vi "Fire Refresh Markers.vi"(8 "error in (no error)":errorcluster, 11 "SequenceViewPanel in":refnum<class "SequenceViewPanel.lvclass">) -> (0 "error out":errorcluster, 3 "SequenceViewPanel out":refnum<class "SequenceViewPanel.lvclass">)   [LabVIEW 2020, in "TSnax UI.lvlib" / "SequenceViewPanel.lvclass"]
uses:
  SequenceViewPanel.lvclass
  SequenceViewPanel.lvclass/SequenceViewPanel.ctl
  3c1a44d5-48fc-4b93-aa61-ebc8600dc4e9.vi
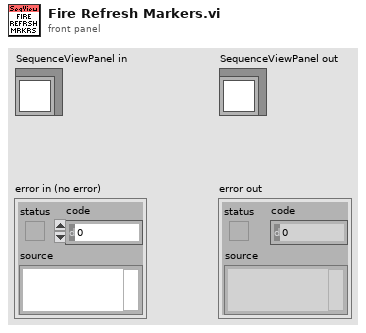
[diagram p1: front panel]
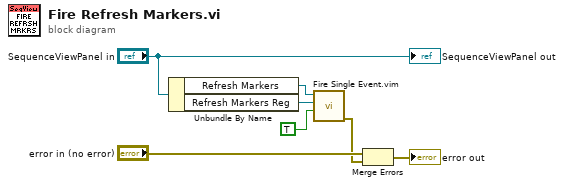
[diagram p0: block diagram]
diagram:
  n1 = Unbundle By Name("SequenceViewPanel in") -> ("Refresh Markers"=w4:refnum<user-event>, "Refresh Markers Reg"=w5:refnum<event-registration>)
  n2 = call "Fire Single Event.vim"("Data"=TRUE ("event data"), "Event Reg"=w5, "Event"=w4) -> ("error out"=w1:errorcluster)  [unwired: 8 in]
  n3 = Merge Errors("error in (no error)", w1) -> (→"error out":errorcluster)
  "SequenceViewPanel out" <- "SequenceViewPanel in"
